vi "get_IP.vi"() -> (2 "IP address":string)   [LabVIEW 2014]
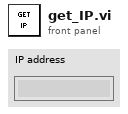
[diagram p1: front panel]
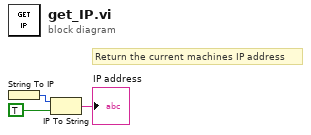
[diagram p0: block diagram]
diagram:
  # "Return the current machines IP address"
  n1 = String To IP() -> (0:w3:u32)  [unwired: 1 in]
  n2 = IP To String(1:TRUE ("dot notation? (F)"), 2:w3) -> (0:→"IP address":string)
